vi "Write Graph-Chart Axis Labels.vi"(8 "error in":errorcluster, 10 "Value":string[](array[string]), 11 "Graph / Chart Reference in":refnum<vi>) -> (0 "error out":errorcluster, 3 "Graph / Chart Reference out":refnum<vi>)   [LabVIEW 2020, in "G-Unicode.lvlib"]
uses:
  G-Unicode.lvlib
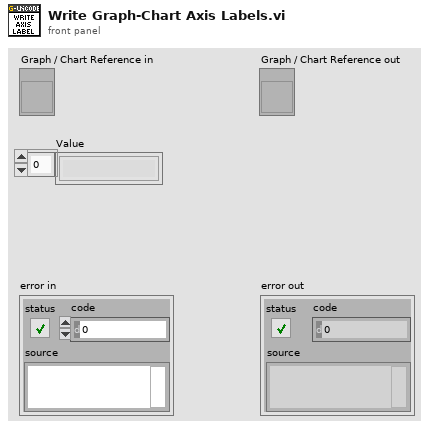
[diagram p1: front panel]
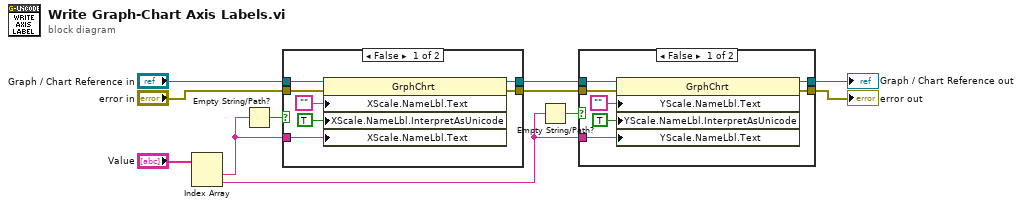
[diagram p0: block diagram]
diagram:
  n1 = Index Array(array="Value") -> (element #1=w4:string, element #2=w2:string)  [unwired: 2 in]
  n2 = Empty String/Path?(string/path=w4) -> (empty?=w3:bool)
  n3 = case shown="False" w3 {
    tunnel: "Graph / Chart Reference in" -> [w16 w20]
    tunnel: "error in" -> [w15 w19]
    tunnel: w4 -> [w14 _]
    tunnel: [w13 w20] -> w8
    tunnel: [w12 w19] -> w6
    frame False {
      n4 = property class="GrphChrt"(reference=w16, error in=w15, "XScale.NameLbl.Text"="" ("Value"), "XScale.NameLbl.InterpretAsUnicode"=TRUE ("Text.Interpret As Unicode"), "XScale.NameLbl.Text"=w14) -> (reference out=w13:refnum<vi>, error out=w12:errorcluster)
    }
    frame True {
    }
  }
  n5 = Empty String/Path?(string/path=w2) -> (empty?=w1:bool)
  n6 = case shown="False" w1 {
    tunnel: w8 -> [w27 w29]
    tunnel: [w26 w29] -> w7
    tunnel: w6 -> [w25 w28]
    tunnel: [w24 w28] -> w5
    tunnel: w2 -> [w23 _]
    frame False {
      n7 = property class="GrphChrt"(reference=w27, error in=w25, "YScale.NameLbl.Text"="" ("Value"), "YScale.NameLbl.InterpretAsUnicode"=TRUE ("Y Scale.Name Label.Interpret As Unicode"), "YScale.NameLbl.Text"=w23) -> (reference out=w26:refnum<vi>, error out=w24:errorcluster)
    }
    frame True {
    }
  }
  "error out" <- w5
  "Graph / Chart Reference out" <- w7
